vi "Error Converter (ErrCode or Status).vi"(8 "error in (no error)":errorcluster, 11 "error code":i32) -> (0 "error out":errorcluster)   [LabVIEW 2013, in "Baseline.lvlib"]
uses:
  <userlib>/Baseline/Baseline.lvlib
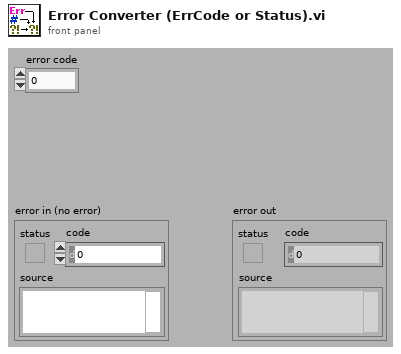
[diagram p1: front panel]
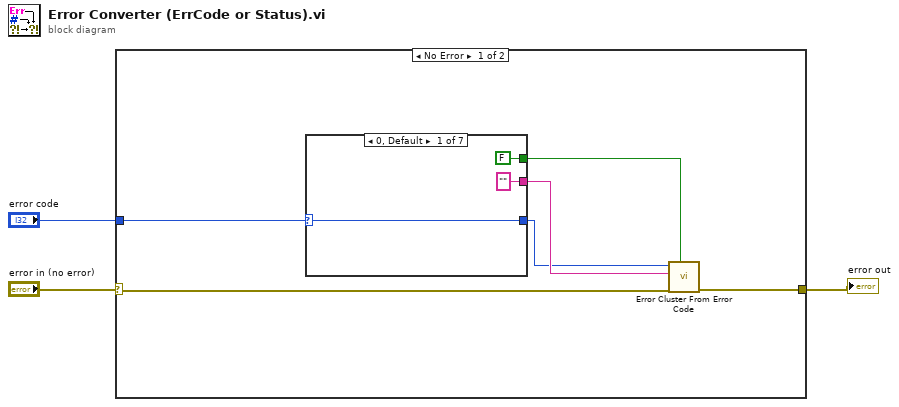
[diagram p0: block diagram]
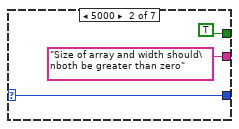
[diagram p2: hidden frame]
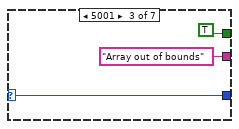
[diagram p3: hidden frame]
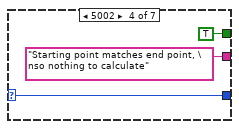
[diagram p4: hidden frame]
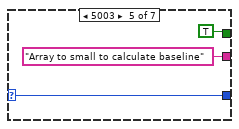
[diagram p5: hidden frame]
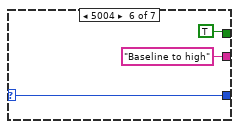
[diagram p6: hidden frame]
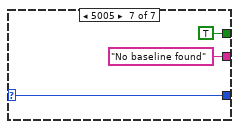
[diagram p7: hidden frame]
diagram:
  n1 = case shown="No Error" "error in (no error)" {
    selector: "error in (no error)" -> [w9 w31]
    tunnel: [w8 w31] -> w2
    tunnel: "error code" -> [w7 _]
    frame No Error {
      n2 = case shown="0, Default" w7 {
        selector: w7 -> [w12 w14 w18 w21 w24 w27 w30]
        tunnel: ["" ("string") "Size of array and width should\nboth be greater than zero" ("string") "Array out of bounds" ("string") "Starting point matches end point, \nso nothing to calculate" ("string") "Array to small to calculate baseline" ("string") "Baseline to high" ("string") "No baseline found" ("string")] -> w6
        tunnel: [w12 w14 w18 w21 w24 w27 w30] -> w5
        tunnel: [FALSE ("show call chain? (False)") TRUE ("show call chain? (False)") TRUE TRUE TRUE TRUE TRUE] -> w4
        frame 0, Default {
        }
        frame 5000 {
        }
        frame 5001 {
        }
        frame 5002 {
        }
        frame 5003 {
        }
        frame 5004 {
        }
        frame 5005 {
        }
      }
      n3 = call <vilib>:"Error Cluster From Error Code.vi"("show call chain? (False)"=w4, "error in (no error)"=w9, "error message (\"\")"=w6, "error code (0)"=w5) -> ("error out"=w8:errorcluster)  [unwired: 5 in]
    }
    frame Error {
    }
  }
  "error out" <- w2
